vi "WriteToRandomFile.vi"() -> ()   [LabVIEW 2026]
panel:
  in  "error in (no error)":errorcluster
  out "error out":errorcluster
  out "text":string
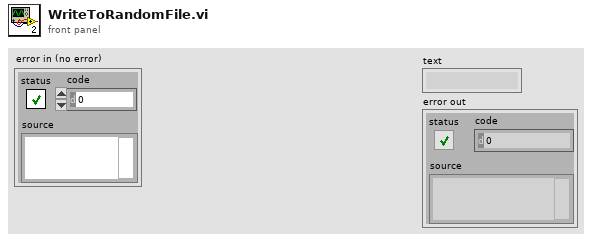
[diagram p1: front panel]
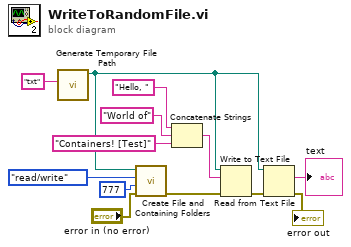
[diagram p0: block diagram]
diagram:
  n1 = call <vilib>:"Generate Temporary File Path.vi"("Temporary File Extension (tmp)"="txt") -> ("Unique Temporary File Path"=w3:path)  [unwired: 9 in, 1 out]
  n2 = call <vilib>:"Create File and Containing Folders.vi"("error in (no error)"="error in (no error)", "permissions"=i16 777, "access"=enum16{"read/write", "read-only", "write-only"}."read/write", "file path"=w3) -> ("error out"=w7:errorcluster)  [unwired: 6 in, 1 out]
  n3 = Concatenate Strings("Hello, " ("string"), "World of" ("string"), "Containers! [Test]" ("string")) -> (w6:string)
  n4 = Write to Text File(file (use dialog)=w3, text=w6, error in=w7) -> (error out=w4:errorcluster)  [unwired: 1 in, 2 out]
  n5 = Read from Text File(file (use dialog)=w3, error in=w4) -> (text=→"text":string, error out=→"error out":errorcluster)  [unwired: 2 in, 2 out]
